vi "TE Signal3.0.vi"() -> ()   [LabVIEW 2010]
doc: "This example illustrates how to use autosetup and acquire multiple waveforms from several channels using the following steps:\n\n1. Specify a valid VISA session. \n2. Specify Channel A. \n3. Specify Channel B.\n4. Specify a time-out value for reading waveform.\n5. Run the VI. The graph displays waveforms you acquire."
uses:
  <vilib>/Platform/storage/lvStorage.llb/xStorage/Open Data Storage/Open Data Storage.xnode
  <vilib>/Platform/storage/lvStorage.llb/_openFunction.ctl
  <vilib>/Platform/storage/lvStorage.llb/xStorage/Set Properties/Set Properties.xnode
  <vilib>/Platform/storage/lvStorage.llb/xStorage/Write Data/Write Data.xnode
  <vilib>/Platform/storage/Storage.llb/usiOverwriteOptions.ctl
  <vilib>/Platform/storage/Storage.llb/usiSequenceRepresentation.ctl
  <vilib>/Platform/storage/lvStorage.llb/xStorage/Close Data Storage/Close Data Storage.xnode
  <instrlib>/Tektronix DPO MSO 2000 4000 Series/Public/Data/Read (Single Waveform).vi
  <instrlib>/Tektronix DPO MSO 2000 4000 Series/Public/Data/Read (Multiple Waveforms).vi
  <instrlib>/Tektronix DPO MSO 2000 4000 Series/Public/Configure/Configure Math (Dual).vi
  <vilib>/Platform/storage/lvStorage.llb/_openStorageWithRootAutoDetect.vi
  <vilib>/Platform/storage/lvStorage.llb/xStorage/xStorageSupp/ErrorOut.vi
  <vilib>/Platform/storage/Storage.llb/__savePropString.vi
  <vilib>/Platform/storage/Storage.llb/__savePropTime.vi
  <vilib>/Platform/storage/Storage.llb/_createExplicitChildObject.vi
  <vilib>/Platform/storage/lvStorage.llb/_prepDDT.vi
  <vilib>/Platform/storage/lvStorage.llb/_getChannelNameFromDDT.vi
  <vilib>/Platform/storage/lvStorage.llb/_saveDDT.vi
  <vilib>/Platform/storage/Storage.llb/Get Object Info.vi
  <vilib>/Platform/storage/Storage.llb/__closeStorageFromObject.vi
  <instrlib>/Tektronix DPO MSO 2000 4000 Series/Tektronix DPO MSO 2000 4000 Series.lvlib
panel:
  out "Averenge":dbl
  out "Periode":dbl
  out "STATUS":string
  in  "Start TEST":bool
  out "?":bool
  out "?":bool
  out "DOWN":dbl
  out "UP":dbl
  in  "Error Range":dbl min=0.0 max=5.0 step=0.1 format="%#.3g"
  out "TIMA":waveform(dbl)(graph)
  out "TIMB":waveform(dbl)(graph)
  in  "Assembled by":string="Alexis Ibarra"
  in  "ABM-S/N":string
  out "Differential Signal":waveform(dbl)(graph)
  in  "Port":u16(ring) items=["AMB 1", "AMB 2", "AMB 3", "AMB 4", "AMB 5", "AMB 18"]
  in  "DPO-4034 IP Adress":string
  out "error out":errorcluster
  in  "Maximum Time (10000ms)":u32=20000
  in  "Channel B (1: Channel 2)":u16(ring)=1 items=["Channel 1", "Channel 2", "Channel 3", "Channel 4", "Math", "Reference 1", "Reference 2", "Reference 3", "Reference 4"]
  in  "Channel A (0: Channel 1)":u16(ring) items=["Channel 1", "Channel 2", "Channel 3", "Channel 4", "Math", "Reference 1", "Reference 2", "Reference 3", "Reference 4"]
  out "TE Signals":waveform(dbl)[](graph)
  # "Actualy ip DPO-4038\n     10.195.18.178"
  # "Select Port"
  # "Error Limit"
  # "ms"
  # "ms"
  # "ms"
  # "Channels"
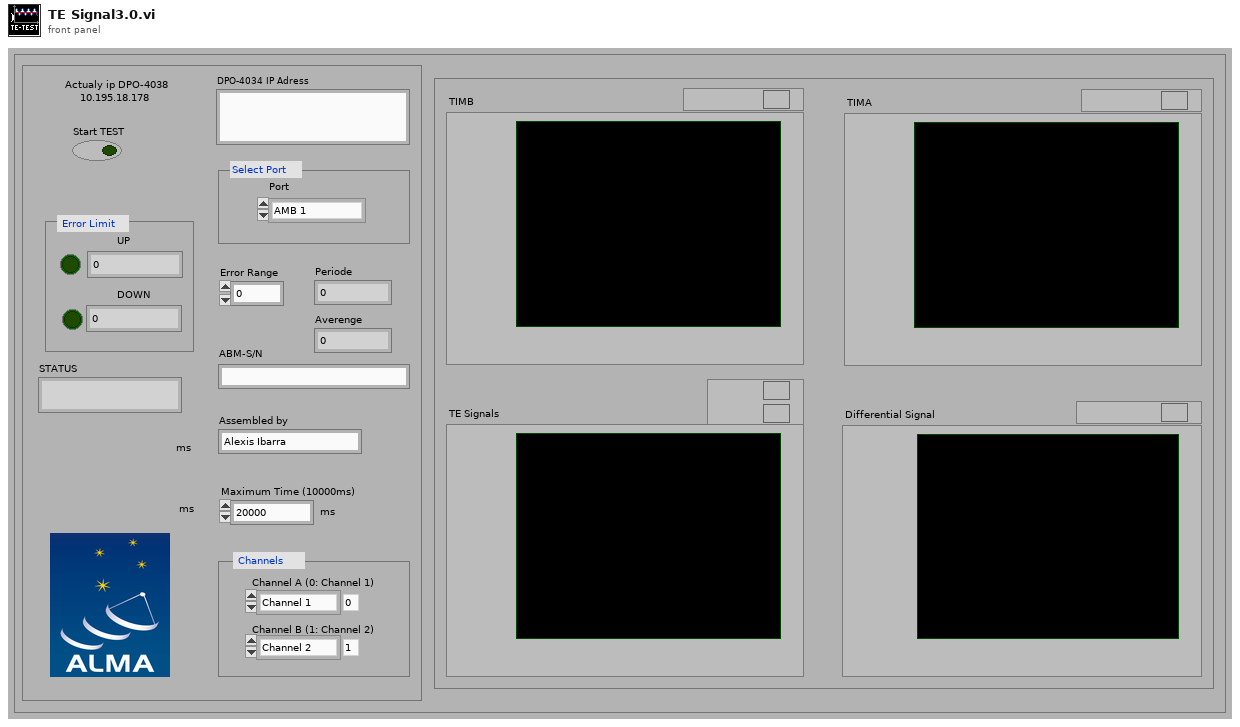
[diagram p1: front panel]
types:
  T1 = enum16{"UPDATE", "READ", "QUERY", "CREATE CHILD", "CREATE", "CONNECT", "DISCONNECT"}
  T2 = typedef "usiOverwriteOptions.ctl" = enum16{"Append values", "Replace values at index", "Replace all values", "Append if timeline aligns"}
  T3 = typedef "usiSequenceRepresentation.ctl" = enum16{"explicit", "implicit"}
  T4 = typedef "_openFunction.ctl" = enum16{"open", "open or create", "create or replace", "create", "open (read only)"}
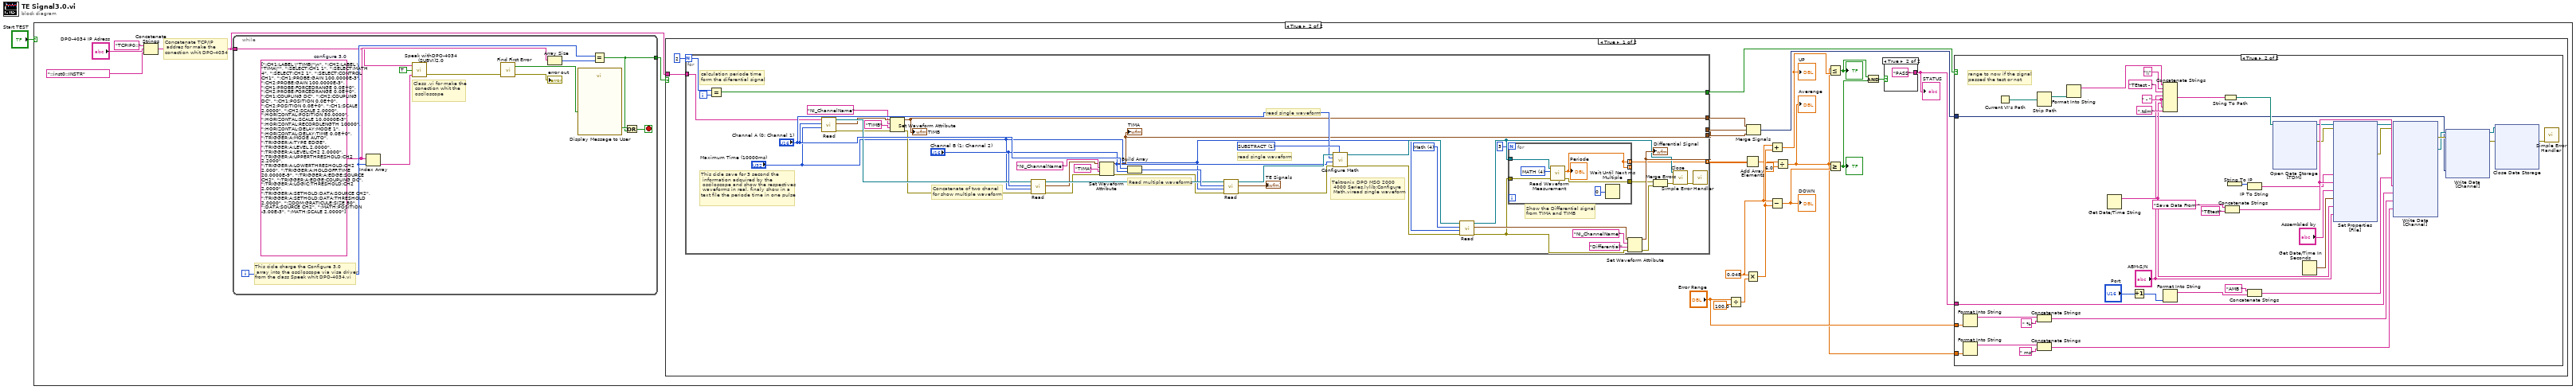
[diagram p0: block diagram]
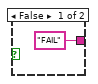
[diagram p3: hidden frame]
diagram:
  n1 = case shown="True" "Start TEST" {
    frame False {
    }
    frame True {
      # "Concatenate TCP/IP\n addres for make the \nconection whit DPO-4034"
      n2 = Concatenate Strings("TCPIP0::", "DPO-4034 IP Adress", "::inst0::INSTR") -> (w2:string)
      n3 = while {
        tunnel: w2 -> [w222]
        tunnel: [w219] -> w3
        i -> [w229]
        stop <- w224 stop-if-true
        w223 = string[] [":CH1:LABEL \"TIMB\"\n", ":CH2:LABEL \"TIMA\"", ":SELECT:CH1 1", ":SELECT:MATH 4", ":SELECT:CH2 1", ":SELECT:CONTROL CH1", ":CH1:PROBE:GAIN 100.0000E-3", ":CH2:PROBE:GAIN 100.0000E-3", ":CH1:PROBE:FORCEDRANGE 0.0E+0", ":CH2:PROBE:FORCEDRANGE 0.0E+0", ":CH1:COUPLING DC", ":CH2:COUPLING DC", ":CH1:POSITION 0.0E+0", ":CH2:POSITION 0.0E+0", ":CH1:SCALE 2.0000", ":CH2:SCALE 2.0000", ":HORIZONTAL:POSITION 50.0000", ":HORIZONTAL:SCALE 10.0000E-3", ":HORIZONTAL:RECORDLENGTH 10000", ":HORIZONTAL:DELAY:MODE 1", ":HORIZONTAL:DELAY:TIME 0.0E+0", ":TRIGGER:A:MODE AUTO", ":TRIGGER:A:TYPE EDGE", ":TRIGGER:A:LEVEL 2.0000", ":TRIGGER:A:LEVEL:CH2 2.0000", ":TRIGGER:A:UPPERTHRESHOLD:CH2 2.2000", ":TRIGGER:A:LOWERTHRESHOLD:CH2 2.000", ":TRIGGER:A:HOLDOFF:TIME 20.0000E-9", ":TRIGGER:A:EDGE:SOURCE CH2", ":TRIGGER:A:EDGE:COUPLING DC", ":TRIGGER:A:LOGIC:THRESHOLD:CH2 2.0000", ":TRIGGER:A:SETHOLD:DATA:SOURCE CH2", ":TRIGGER:A:SETHOLD:DATA:THRESHOLD 2.0000", ":ZOOM:GRATICULE:SIZE 80", ":DATA:SOURCE CH2", ":MATH:POSITION -3.00E-3", ":MATH:SCALE 2.0000"]  # configure 3.0
        # "Class .vi for make the\n conection whit the\n osciloscope"
        # "This cicle charge the Configure 3.0\n array into the osciloscope via visa driver \nfrom the class Speek whit DPO-4034.vi"
        n4 = Index Array "Index Array"(array=w223, index=w229) -> (element=w230:string)
        n5 = call "Speak withDPO-4034 (SUBVI)2.0.vi"("Send Command"=w230, "Send:  TRUE\nRecive: FALSE"=TRUE, "VISA Resource Name"=w222) -> ("error out"=w226:errorcluster)  [unwired: 1 out]
        n6 = call <vilib>:"Find First Error.vi"("error in (no error)"=w226) -> ("error out"=→"error out":errorcluster, "error?"=w220:bool)  [unwired: 3 in]
        n7 = Array Size(array=w223) -> (size(s)=w228:i32)
        n8 = call "Display Message to User"("Enable"=w220) -> ("OK"=w221:bool)  [unwired: 9 in, 1 out]
        n9 = Equal?(x=w229, y=w228) -> (x = y?=w219:bool)
        n10 = Or(x=w221, y=w219) -> (x .or. y?=w224:bool)
      }
      n11 = case shown="True" w3 {
        tunnel: w2 -> [w28 _]
        frame True {
          w24 = 0.048 ("x")
          n12 = for {
            N: 2 -> [w32]
            tunnel: [w43] -> w16
            tunnel: w28 -> [w58]
            tunnel: [w55] -> w14
            tunnel: [w47] -> w15
            tunnel: [w31] -> w27
            tunnel: [w29] -> w10 mode=indexing
            i -> [w33]
            w39 = u16 4 items=["Channel 1", "Channel 2", "Channel 3", "Channel 4", "Math", "Reference 1", "Reference 2", "Reference 3", "Reference 4"] ("Channel (0: Channel 1)")
            w66 = u16 1 items=["ADD", "SUBSTRACT", "MULTIPLY", "DIVIDE"] ("Operator (0: ADD)")
            # "This cicle save for 3 second the\n information adquired by the\n osciloscope and show the respectives\n waveforms in real, finaly show in a \ntext file the periode time in one pulse"
            # "Concatenate of two chanel \nfor show multiple waveform"
            # "read single waveform"
            # "read single waveform"
            # "Tektronix DPO MSO 2000\n 4000 Series.lvlib:Configure\n Math.viread single waveform"
            # "calculation periode time\nform the diferential signal"
            # "Show the Differential signal \nfrom TIMA and TIMB"
            # "Read multiple waveforms"
            n13 = Equal?(x=w32, y=w33) -> (x = y?=w31:bool)
            n14 = call-poly <instrlib>:"Read.vi"("Maximum Time (10000ms)"="Maximum Time (10000ms)", "Channel (0: Channel 1)"="Channel A (0: Channel 1)", "VISA resource name"=w58) -> ("error out"=w54:errorcluster, "Waveform Graph"=w57:waveform(dbl), "VISA resource name out"=w60:refnum<visa-resource-name>)  [unwired: 6 in]
            n15 = Set Waveform Attribute(4:w54, 5:"TIMB" ("name"), 6:"NI_ChannelName" ("name"), 7:w57) -> (0:w53:errorcluster, 3:w55:waveform(dbl))  [unwired: 1 out]
            "TIMB" <- w55
            n16 = call-poly <instrlib>:"Read.vi"("error in (no error)"=w53, "Maximum Time (10000ms)"="Maximum Time (10000ms)", "Channel (0: Channel 1)"="Channel B (1: Channel 2)", "VISA resource name"=w60) -> ("error out"=w49:errorcluster, "Waveform Graph"=w50:waveform(dbl), "VISA resource name out"=w59:refnum<visa-resource-name>)  [unwired: 5 in]
            n17 = Set Waveform Attribute(4:w49, 5:"TIMA" ("name"), 6:"NI_ChannelName" ("name"), 7:w50) -> (0:w48:errorcluster, 3:w47:waveform(dbl))  [unwired: 1 out]
            "TIMA" <- w47
            n18 = Build Array("Channel A (0: Channel 1)", "Channel B (1: Channel 2)") -> (w68:u16[])
            n19 = call-poly <instrlib>:"Read.vi"("error in (no error)"=w48, "Maximum Time (10000ms)"="Maximum Time (10000ms)", "Channels"=w68, "VISA resource name"=w59) -> ("error out"=w67:errorcluster, "Waveform Data"=→"TE Signals":waveform(dbl)[], "VISA resource name out"=w64:refnum<visa-resource-name>)  [unwired: 5 in]
            n20 = call-poly <instrlib>:"Configure Math.vi"("Operator (0: ADD)"=w66, "error in (no error)"=w67, "2nd Source (1: Channel 2)"="Channel B (1: Channel 2)", "1st Source (0: Channel 1)"="Channel A (0: Channel 1)", "VISA resource name"=w64) -> ("error out"=w63:errorcluster, "VISA resource name out"=w65:refnum<visa-resource-name>)  [unwired: 5 in]
            n21 = call-poly <instrlib>:"Read.vi"("error in (no error)"=w63, "Maximum Time (10000ms)"="Maximum Time (10000ms)", "Channel (0: Channel 1)"=w39, "VISA resource name"=w65) -> ("error out"=w37:errorcluster, "Waveform Graph"=w44:waveform(dbl), "VISA resource name out"=w38:refnum<visa-resource-name>)  [unwired: 5 in]
            n22 = for {
              N: 3 -> [_]
              tunnel: w38 -> [w75]
              tunnel: w37 -> [w73]
              tunnel: [w71] -> w36
              tunnel: [w70] -> _ mode=indexing
              tunnel: [w70] -> w29 mode=indexing
              w74 = u16 4 items=["Channel 1", "Channel 2", "Channel 3", "Channel 4", "MATH", "Reference 1", "Reference 2", "Reference 3", "Reference 4"] ("Channel (0: Channel 1)")
              n23 = call <instrlib>:"Read Waveform Measurement.vi"("error in (no error)"=w73, "Channel (0: Channel 1)"=w74, "VISA resource name"=w75) -> ("error out"=w71:errorcluster, "Measurement Value"=w70:dbl)  [unwired: 6 in, 1 out]
              "Periode" <- w70
              n24 = Wait Until Next ms Multiple(millisecond multiple=u32 0) -> ()  [unwired: 1 out]
            }
            n25 = Set Waveform Attribute(4:w37, 5:"Differential" ("name"), 6:"NI_ChannelName" ("name"), 7:w44) -> (0:w35:errorcluster, 3:w43:waveform(dbl))  [unwired: 1 out]
            "Differential Signal" <- w43
            n26 = Merge Errors(w36, w35) -> (w34:errorcluster)
            n27 = call <instrlib>:"Close.vi"("error in (no error)"=w34, "VISA resource name"=w38) -> ("error out"=w69:errorcluster)  [unwired: 9 in]
            n28 = call <vilib>:"Simple Error Handler.vi"("error in (no error)"=w69) -> ()  [unwired: 4 in, 5 out]
          }
          n29 = Divide(x="Error Range", y=100.0) -> (x/y=w25:dbl)
          n30 = Add Array Elements(numeric array=w10) -> (sum=w9:dbl)
          n31 = Multiply(x=w24, y=w25) -> (x*y=w23:dbl)
          n32 = Merge Signals "Merge Signals"(w14, w15, w16) -> (w13:dynamicdata)
          n33 = Add(x=w24, y=w23) -> (x+y=w21:dbl)
          "UP" <- w21
          n34 = Subtract(x=w24, y=w23) -> (x-y=w20:dbl)
          "DOWN" <- w20
          n35 = Divide(x=w9, y=6.0) -> (x/y=w7:dbl)
          "Averenge" <- w7
          n36 = Less Or Equal?(x=w7, y=w21) -> (x <= y?=w19:bool)
          "?" <- w19
          n37 = Greater Or Equal?(x=w7, y=w20) -> (x >= y?=w18:bool)
          "?" <- w18
          n38 = And(x=w19, y=w18) -> (x .and. y?=w22:bool)
          n39 = case shown="True" w22 {
            tunnel: ["FAIL" "PASS"] -> w12
            frame False {
            }
            frame True {
            }
          }
          "STATUS" <- w12
          n40 = case shown="True" w27 {
            tunnel: w7 -> [_ w81]
            tunnel: "Error Range" -> [_ w80]
            tunnel: w12 -> [_ w79]
            tunnel: w13 -> [_ w78]
            frame False {
            }
            frame True {
              w102 = " - " ("string")
              # "range to now if the signal\npassed the test or not"
              n41 = Format Into String "Format Into String"(w80) -> (resulting string=w107:string)  [unwired: 3 in, 1 out]
              n42 = Format Into String "Format Into String"(w81) -> (resulting string=w105:string)  [unwired: 3 in, 1 out]
              n43 = Current VI's Path() -> (path=w88:path)
              n44 = Strip Path(path=w88) -> (stripped path=w87:path)  [unwired: 1 out]
              n45 = Concatenate Strings "Concatenate Strings"(w107, " %") -> (w117:string)
              n46 = Concatenate Strings "Concatenate Strings"(w105, " ms") -> (w118:string)
              n47 = Format Into String "Format Into String"(w87) -> (resulting string=w89:string)  [unwired: 3 in, 1 out]
              n48 = Get Date/Time String() -> (date string=w101:string)  [unwired: 3 in, 1 out]
              n49 = Increment(x="Port") -> (x+1=w104:u16)
              n50 = Concatenate Strings "Concatenate Strings"(w89, "\\", "TEtest - " ("string"), "ABM-S/N", w102, w101, w102, ".tdm") -> (w85:string)
              n51 = Format Into String "Format Into String"(w104) -> (resulting string=w111:string)  [unwired: 3 in, 1 out]
              n52 = String To Path(string=w85) -> (path=w84:path)
              n53 = Concatenate Strings "Concatenate Strings"("Save Data From ", "TEtest") -> (w119:string)
              n54 = String To IP() -> (0:w95:u32)  [unwired: 1 in]
              n55 = IP To String(2:w95) -> (0:w94:string)  [unwired: 1 in]
              n56 = Concatenate Strings "Concatenate Strings"("AMB ", w111) -> (w114:string)
              n57 = xnode "Open Data Storage\n[TDM]"("file path"=w84) -> ("storage refnum (file)"=w91:refnum<k20>, "error out"=w110:errorcluster)  [unwired: 4 in, 1 out]
              n58 = Get Date/Time In Seconds() -> (seconds since 1Jan1904=w90:timestamp)
              n59 = xnode "Set Properties\n[File]"("Name"=w94, "Description"=w119, "Author"="Assembled by", "Time stamp"=w90, "Date"=w101, "ABM_SerialNumber"="ABM-S/N", "storage refnum (file)"=w91, "error in"=w110) -> ("storage refnum (file) out"=w112:refnum<k20>, "error out"=w113:errorcluster)
              n60 = xnode "Write Data\n[Channel]"("Name"=w114, "Description"=w119, "Status"=w79, "Error_Range"=w117, "Periode"=w118, "storage refnum (file)"=w112, "error in"=w113) -> ("error out"=w116:errorcluster, "storage refnum (channel group)"=w115:refnum<k20>)  [unwired: 1 out]
              n61 = xnode "Write Data\n[Channel]"("Signal"=w78, "storage refnum (channel group)"=w115, "error in"=w116) -> ("storage refnum (channel group) out"=w97:refnum<k20>, "error out"=w98:errorcluster)  [unwired: 2 in, 1 out]
              n62 = xnode "Close Data Storage\n"("storage refnum (channel group)"=w97, "error in (no error)"=w98) -> ("error out"=w96:errorcluster)  [unwired: 1 out]
              n63 = call <vilib>:"Simple Error Handler.vi"("error in (no error)"=w96) -> ()  [unwired: 1 in, 8 out]
            }
          }
        }
        frame False {
        }
      }
    }
  }
